vi "Nov_26.vi"() -> ()   [LabVIEW 2020]
panel:
  out "Acc X - Right":dynamicdata(graph)
  out "Signal Filtered":dynamicdata(graph)
  out "Swing":bool
  in  "Record Signal":bool
  in  "STOP":bool
  # "Gait Events"
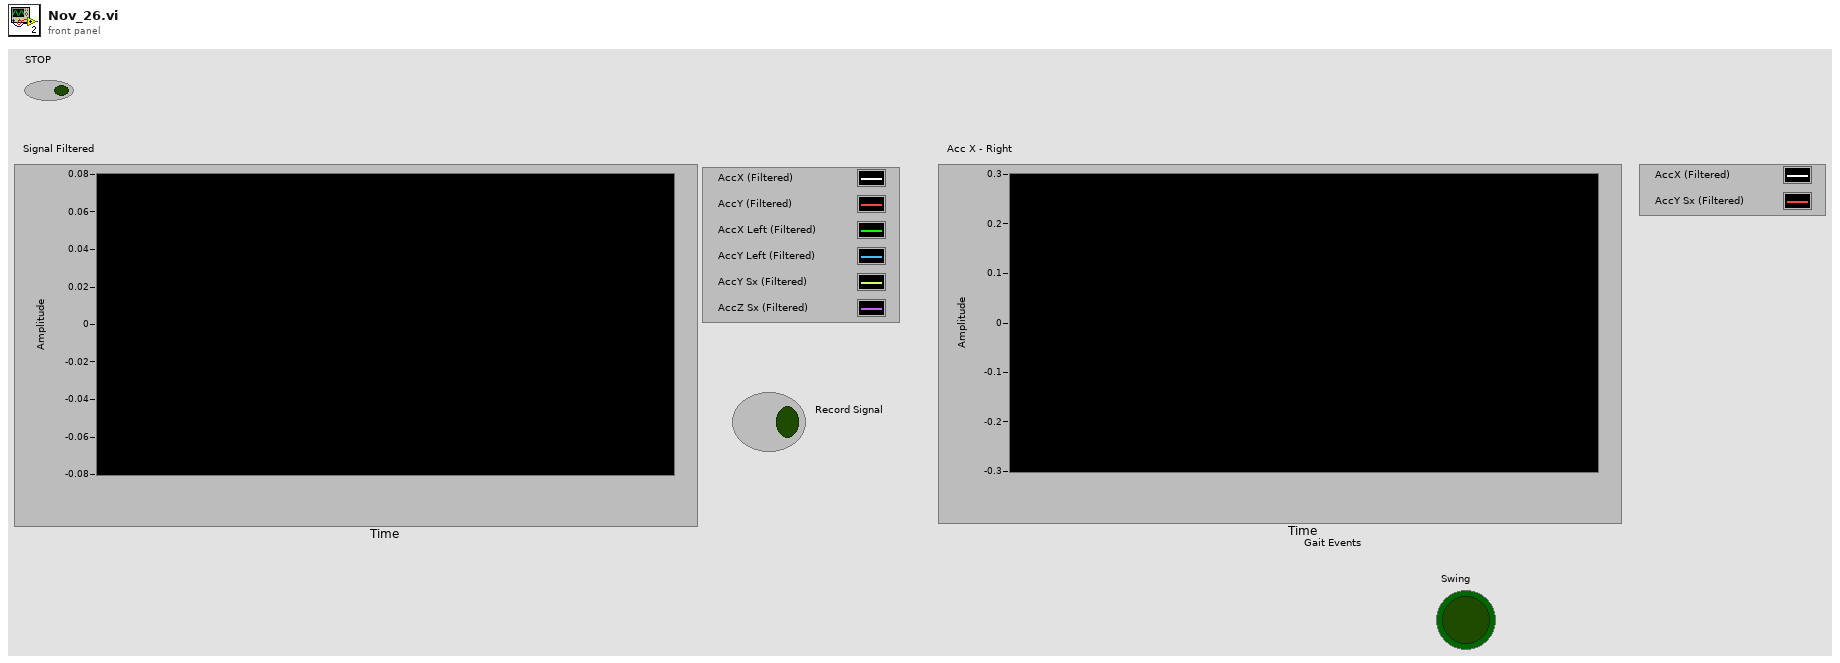
[diagram p1: front panel]
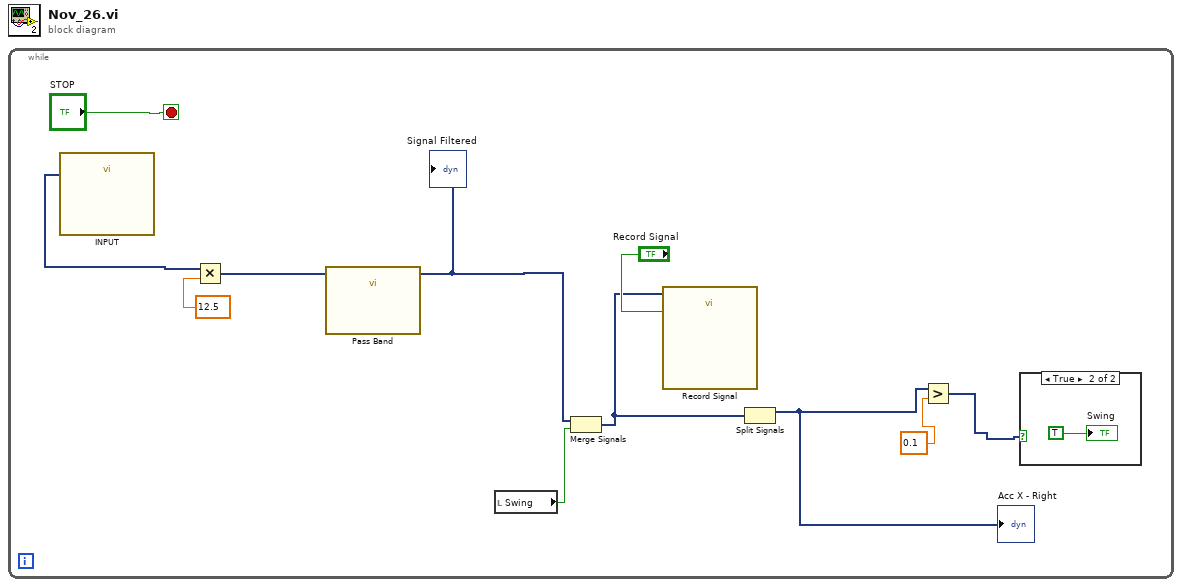
[diagram p0: block diagram]
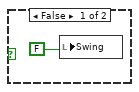
[diagram p2: hidden frame]
diagram:
  n1 = while {
    stop <- "STOP" stop-if-true
    n2 = call "INPUT"() -> ("data"=w2:dynamicdata)  [unwired: 16 in, 3 out]
    n3 = Multiply(x=w2, y=12.5) -> (x*y=w6:dynamicdata)
    n4 = call "Pass Band"("Signal"=w6) -> ("Filtered Signal"=w9:dynamicdata)  [unwired: 9 in, 1 out]
    "Signal Filtered" <- w9
    n5 = local read "Swing"() -> (w1:bool)
    n6 = Merge Signals(w9, w1) -> (w8:dynamicdata)
    n7 = call "Record Signal"("Signals"=w8, "Enable"="Record Signal") -> ()  [unwired: 15 in, 3 out]
    n8 = Split Signals(w8) -> (w3:dynamicdata)  [unwired: 2 in, 1 out]
    "Acc X - Right" <- w3
    n9 = Greater?(x=w3, y=0.1) -> (0:w4:dynamicdata)
    n10 = case shown="True" w4 {
      frame False {
        n11 = local write "Swing"(FALSE) -> ()
      }
      frame True {
        "Swing" <- TRUE
      }
    }
  }
